vi "期末-6.vi"() -> ()   [LabVIEW 2014]
uses:
  <vilib>/vision/NI_Vision_Development_Module.lvlib
panel:
  in  "紀錄":bool
  out "分量和":dbl[](array[numeric])
  in  "填入飽和磁場分量中點座標":dbl[](array[numeric])
  in  "Stop Button":bool
  out "0. 原始畫面":T1(plugin-control)
  in  "1. 範圍選擇":T2={"色相（H）"={0, 255}, "飽和度（S）"={0, 255}, "亮度（L）"={0, 255}} {"亮度（L）" scale=0.0..255.0; "飽和度（S）" scale=0.0..255.0; "色相（H）" scale=0.0..255.0}
  out "Number of Particles":i32
  out "output cluster":cluster{"X":dbl, "Y":dbl}
  in  "顏色範圍初始化":bool
  in  "Tab Control":T3(tab)
  out "1. 顏色選取":T1(plugin-control)
  out "2. 填補空隙":T1(plugin-control)
  out "4. 形狀修正":T1(plugin-control)
  out "5. 選取結果":T1(plugin-control)
  out "Particle Measurements":dbl[][](array[numeric])
  out "Error Out":errorcluster
  out "瞬間尖點座標":dbl[][](array[numeric])
  out "滑鼠位置顏色":T4
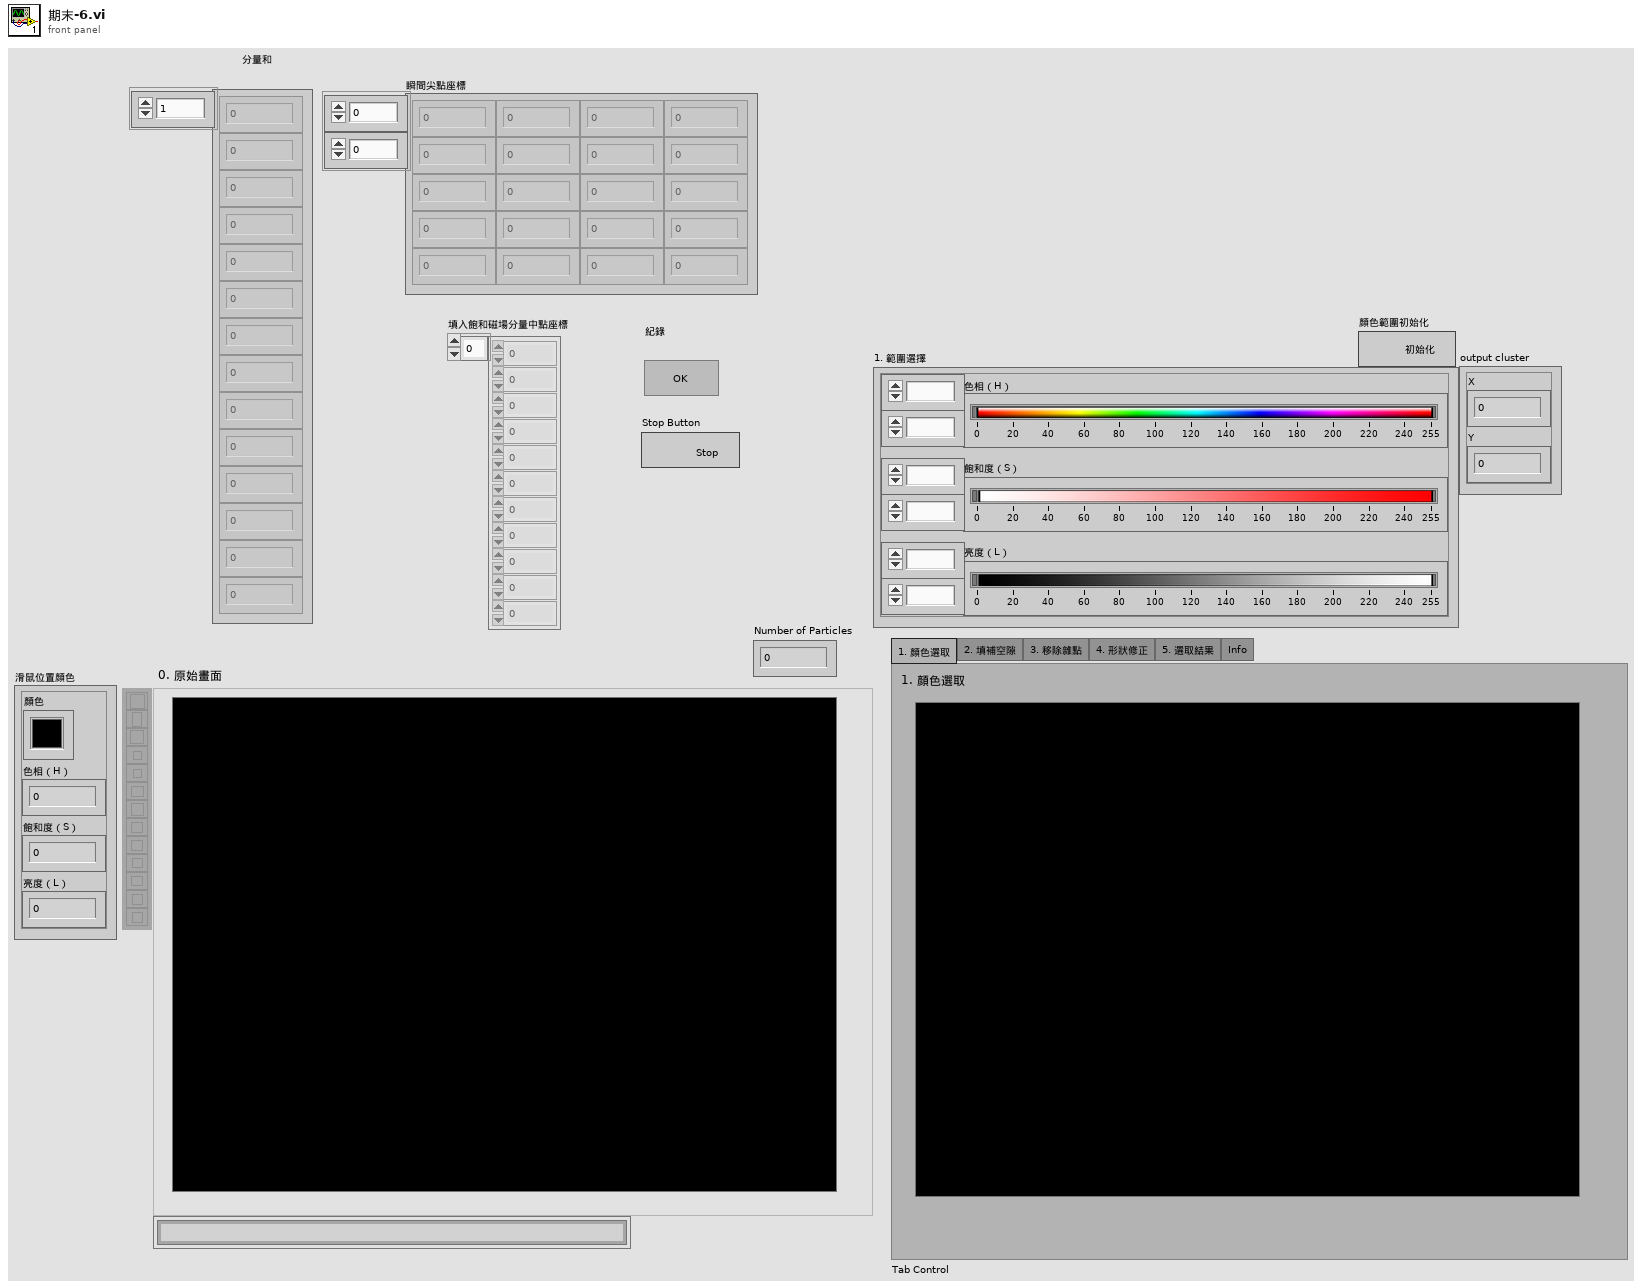
[diagram p1: front panel]
types:
  T1 = typedef "IMAQ Image.ctl" = refnum<image>
  T2 = cluster{"色相（H）":cluster{u8, u8}, "飽和度（S）":cluster{u8, u8}, "亮度（L）":cluster{u8, u8}}
  T3 = enum32{"1. 顏色選取", "2. 填補空隙", "3. 移除雜點", "4. 形狀修正", "5. 選取結果", "Info"}
  T4 = cluster{"色相（H）":u8, "飽和度（S）":u8, "亮度（L）":u8, "顏色":u32}
  T5 = cluster{"Numeric":dbl, "Numeric":dbl, "Numeric":dbl, "Numeric":dbl}
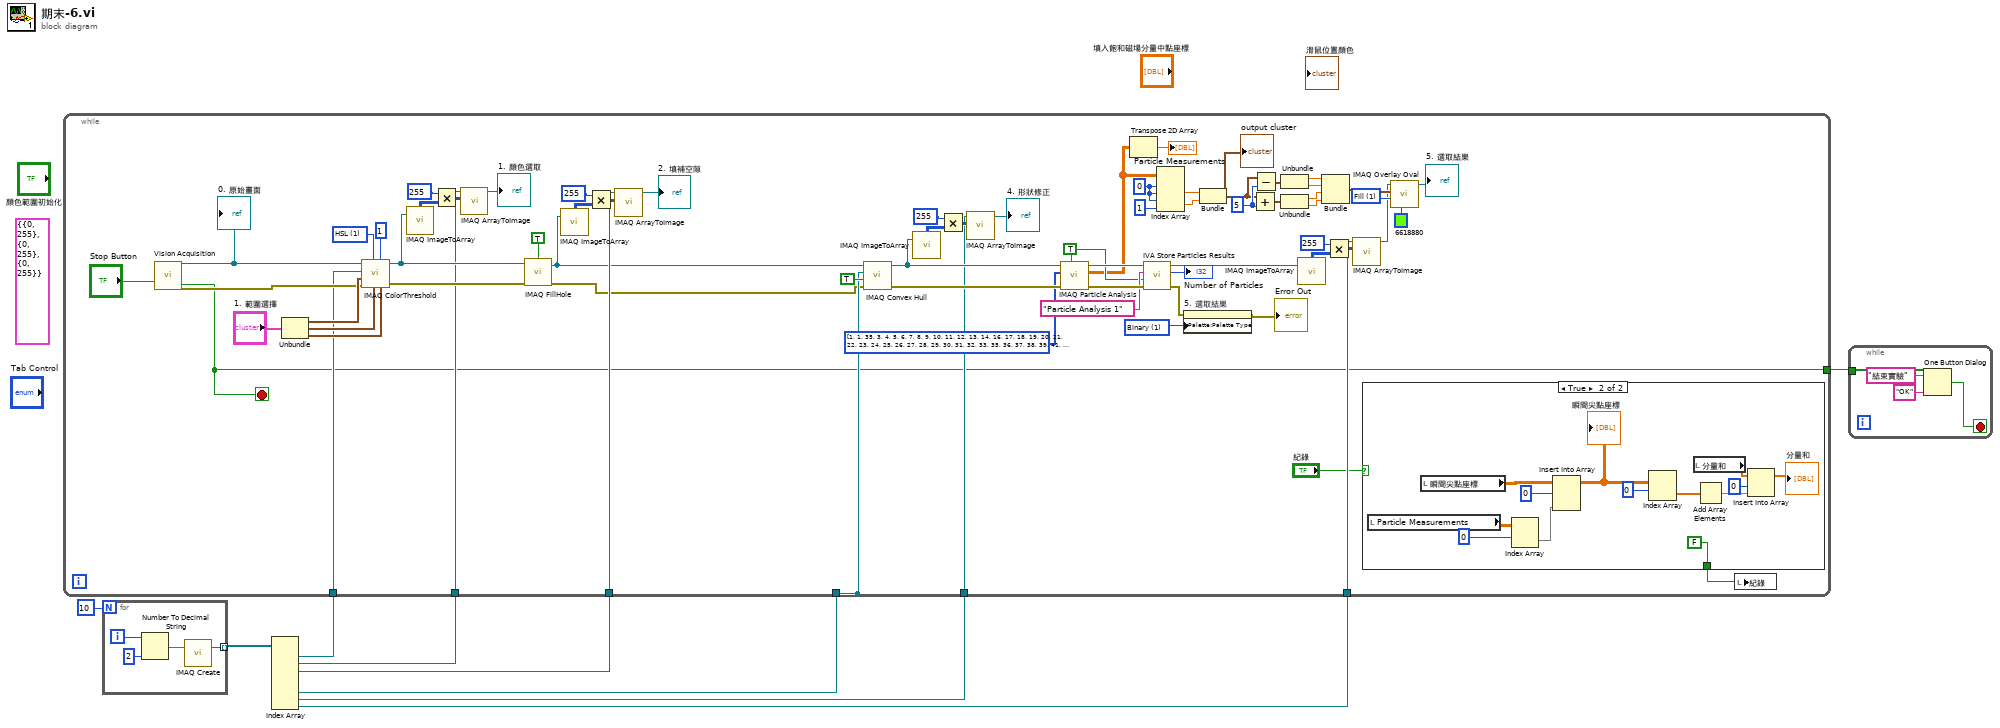
[diagram p0: block diagram]
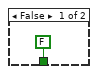
[diagram p2: hidden frame]
diagram:
  (unwired) T2 {"色相（H）"={0, 255}, "飽和度（S）"={0, 255}, "亮度（L）"={0, 255}} ("範圍選擇")
  n1 = for {
    N: 10 -> [_]
    tunnel: [w10] -> w9 mode=indexing
    i -> [w12]
    n2 = Number To Decimal String(number=w12, width (-)=2) -> (decimal integer string=w11:string)
    n3 = call "IMAQ Create"("Image Name"=w11) -> ("New Image"=w10:T1)  [unwired: 4 in, 1 out]
  }
  n4 = Index Array(array=w9) -> (element #1=w8:T1, element #2=w7:T1, element #3=w6:T1, element #6=w4:T1, element #7=w3:T1, element #8=w2:T1)  [unwired: 8 in, 2 out]
  n5 = while {
    tunnel: w6 -> [w52]
    tunnel: w4 -> [w63]
    tunnel: [w63] -> _
    tunnel: w7 -> [w57]
    tunnel: w8 -> [w51]
    tunnel: w3 -> [w45]
    tunnel: w2 -> [w22]
    tunnel: [w16] -> w1
    stop <- w16 stop-if-true
    w27 = u32 1 items=["Frame", "Fill"] ("Drawing Mode (Frame)")
    w36 = 5
    w41 = 0
    w65 = u32 1 items=["Grayscale", "Binary", "Gradient", "Rainbow", "Temperature", "User Defined"] ("Palette")
    w70 = i32[] [1, 1, 35, 3, 4, 5, 6, 7, 8, 9, 10, 11, 12, 13, 14, 16, 17, 18, 19, 20, 21, 22, 23, 24, 25, 26, 27, 28, 29, 30, 31, 32, 33, 35, 36, 37, 38, 39, 41, 42, 43, 45, 46, 48, 49, 50, 51, 53, 54, 55, 56, 58, 59, 60, 61, 62, 63, 64, 65, 66, 68, 69, 70, 71, 72, 73, 74, 75, 76, 77, 78, 79, 80, 81, 82, 83, 84, 85, 86, 87, 88] items=["Center of Mass X", "Center of Mass Y", "First Pixel X", "First Pixel Y", "Bounding Rect Left", "Bounding Rect Top", "Bounding Rect Right", "Bounding Rect Bottom", "Max Feret Diameter Start X", "Max Feret Diameter Start Y", "Max Feret Diameter End X", "Max Feret Diameter End Y", "Max Horiz. Segment Length Left", "Max Horiz. Segment Length Right", "Max Horiz. Segment Length Row", "-", "Bounding Rect Width", "Bounding Rect Height", "Bounding Rect Diagonal", "Perimeter", "Convex Hull Perimeter", "Holes' Perimeter", "Max Feret Diameter", "Equivalent Ellipse Major Axis", "Equivalent Ellipse Minor Axis", "Equivalent Ellipse Minor Axis (Feret)", "Equivalent Rect Long Side", "Equivalent Rect Short Side", "Equivalent Rect Diagonal", "Equivalent Rect Short Side (Feret)", "Average Horiz. Segment Length", "Average Vert. Segment Length", "Hydraulic Radius", "Waddel Disk Diameter", "-", "Area", "Holes' Area", "Particle & Holes' Area", "Convex Hull Area", "Image Area", "-", "Number of Holes", "Number of Horiz. Segments", "Number of Vert. Segments", "-", "Orientation", "Max Feret Diameter Orientation", "-", "% Area/Image Area", "% Area/(Particle & Holes' Area)", "Ratio of Equivalent Ellipse Axes", "Ratio of Equivalent Rect Sides", "-", "Elongation Factor", "Compactness Factor", "Heywood Circularity Factor", "Type Factor", "-", "Sum X", "Sum Y", "Sum XX", "Sum XY", "Sum YY", "Sum XXX", "Sum XXY", "Sum XYY", "Sum YYY", "-", "Moment of Inertia XX", "Moment of Inertia XY", "Moment of Inertia YY", "Moment of Inertia XXX", "Moment of Inertia XXY", "Moment of Inertia XYY", "Moment of Inertia YYY", "Norm. Moment of Inertia XX", "Norm. Moment of Inertia XY", "Norm. Moment of Inertia YY", "Norm. Moment of Inertia XXX", "Norm. Moment of Inertia XXY", "Norm. Moment of Inertia XYY", "Norm. Moment of Inertia YYY", "Hu Moment 1", "Hu Moment 2", "Hu Moment 3", "Hu Moment 4", "Hu Moment 5", "Hu Moment 6", "Hu Moment 7"] ("Pixel Measurements")
    w72 = TRUE ("Connectivity 4/8 (8)")
    w81 = u16 1 items=["RGB", "HSL", "HSV", "HSI"] ("Color Mode")
    n6 = call "Vision Acquisition"("Stop (F)"="Stop Button") -> ("Image Out"=w83:T1, "Stopped"=w16:bool, "error out"=w76:errorcluster)  [unwired: 24 in]
    "0. 原始畫面" <- w83
    n7 = Unbundle("1. 範圍選擇") -> ("色相（H）"=w80:cluster{u8, u8}, "飽和度（S）"=w79:cluster{u8, u8}, "亮度（L）"=w78:cluster{u8, u8})
    n8 = call "IMAQ ColorThreshold"("Blue or Luma or Val or Inten Range"=w78, "Replace Value"=1, "Green or Sat Range"=w79, "Color Mode"=w81, "error in (no error)"=w76, "Red or Hue Range"=w80, "Image Dst"=w51, "Image Src"=w83) -> ("error out"=w67:errorcluster, "Image Dst Out"=w62:T1)  [unwired: 2 out]
    n9 = call "IMAQ ImageToArray"("Image"=w62) -> ("Image Pixels (U8)"=w60:u8[][])  [unwired: 3 in, 4 out]
    n10 = Multiply(x=255, y=w60) -> (x*y=w59:i32[][])
    n11 = call "IMAQ ArrayToImage"("Image Pixels (U8)"=w59, "Image"=w57) -> ("Image Out"=→"1. 顏色選取":T1)  [unwired: 8 in, 1 out]
    n12 = call "IMAQ FillHole"("error in (no error)"=w67, "Image Src"=w62, "Connectivity 4/8 (8)"=TRUE) -> ("error out"=w14:errorcluster, "Image Dst Out"=w15:T1)  [unwired: 1 in, 2 out]
    n13 = call "IMAQ ImageToArray"("Image"=w15) -> ("Image Pixels (U8)"=w55:u8[][])  [unwired: 3 in, 4 out]
    n14 = Multiply(x=255, y=w55) -> (x*y=w56:i32[][])
    n15 = call "IMAQ ArrayToImage"("Image Pixels (U8)"=w56, "Image"=w52) -> ("Image Out"=→"2. 填補空隙":T1)  [unwired: 8 in, 1 out]
    n16 = call "IMAQ Convex Hull"("error in (no error)"=w14, "Connectivity 4/8 (8)"=TRUE, "Image Dst"=w63, "Image Src"=w15) -> ("error out"=w71:errorcluster, "Image Dst Out"=w46:T1)  [unwired: 6 out]
    n17 = call "IMAQ ImageToArray"("Image"=w46) -> ("Image Pixels (U8)"=w49:u8[][])  [unwired: 3 in, 4 out]
    n18 = Multiply(x=255, y=w49) -> (x*y=w50:i32[][])
    n19 = call "IMAQ ArrayToImage"("Image Pixels (U8)"=w50, "Image"=w45) -> ("Image Out"=→"4. 形狀修正":T1)  [unwired: 8 in, 1 out]
    n20 = call "IMAQ Particle Analysis"("Connectivity 4/8 (8)"=w72, "error in (no error)"=w71, "Pixel Measurements"=w70, "Image"=w46) -> ("error out"=w75:errorcluster, "Particle Measurements (Pixels)"=w42:dbl[][], "Image Out (duplicate)"=w73:T1)  [unwired: 1 in, 4 out]
    n21 = Transpose 2D Array(2D array=w42) -> (transposed array=→"Particle Measurements":dbl[][])
    n22 = call <vilib>:"IVA Store Particles Results.vi"("error in (no error)"=w75, "Connectivity 4/8 (8)"=w72, "Step Name"="Particle Analysis 1", "Image in"=w73) -> ("error out"=w66:errorcluster, "Number of Particles"=→"Number of Particles":i32, "Image dup"=w26:T1)  [unwired: 5 out]
    n23 = Index Array(array=w42, index (row) #1=w41, index (col) #1=w41, index (row) #2=w41, index (col) #2=1) -> (element #1=w39:dbl, element #2=w38:dbl)
    n24 = property on="5. 選取結果" class="ImageControl"(error in=w66, "Palette:Palette Type"=w65) -> (error out=→"Error Out":errorcluster)  [unwired: 1 in, 1 out]
    n25 = Bundle("Numeric"=w39, "Numeric"=w38) -> (w35:cluster{"Numeric":dbl, "Numeric":dbl})  [unwired: 1 in]
    "output cluster" <- w35
    n26 = Add(x=w35, y=w36) -> (x+y=w33:cluster{"Numeric":dbl, "Numeric":dbl})
    n27 = Subtract(x=w35, y=w36) -> (x-y=w34:cluster{"Numeric":dbl, "Numeric":dbl})
    n28 = Unbundle(w34) -> ("Numeric"=w32:dbl, "Numeric"=w31:dbl)
    n29 = Unbundle(w33) -> ("Numeric"=w30:dbl, "Numeric"=w29:dbl)
    n30 = call "IMAQ ImageToArray"("Image"=w26) -> ("Image Pixels (U8)"=w23:u8[][])  [unwired: 3 in, 4 out]
    n31 = Bundle("Numeric"=w32, "Numeric"=w31, "Numeric"=w30, "Numeric"=w29) -> (w28:T5)  [unwired: 1 in]
    n32 = Multiply(x=255, y=w23) -> (x*y=w24:i32[][])
    n33 = call "IMAQ ArrayToImage"("Image Pixels (U8)"=w24, "Image"=w22) -> ("Image Out"=w21:T1)  [unwired: 8 in, 1 out]
    n34 = case shown="True" "紀錄" {
      tunnel: [FALSE FALSE] -> w17
      frame False {
      }
      frame True {
        n35 = local read "Particle Measurements"() -> (w87:dbl[][])
        n36 = local read "瞬間尖點座標"() -> (w93:dbl[][])
        n37 = Index Array(array=w87, index (row)=0) -> (element=w92:dbl[])  [unwired: 1 in]
        n38 = Insert Into Array(array=w93, index (row)=0 ("index"), new element=w92) -> (w95:dbl[][])  [unwired: 1 in]
        "瞬間尖點座標" <- w95
        n39 = Index Array(array=w95, index (row)=0) -> (element=w97:dbl[])  [unwired: 1 in]
        n40 = local read "分量和"() -> (w88:dbl[])
        n41 = Add Array Elements(numeric array=w97) -> (sum=w90:dbl)
        n42 = Insert Into Array(array=w88, index=0 ("index (row)"), new element=w90) -> (→"分量和":dbl[])
      }
    }
    n43 = call "IMAQ Overlay Oval"("Color"=u32 6618880, "Drawing Mode (Frame)"=w27, "Bounding Rectangle"=w28, "Image"=w21) -> ("Image Out"=→"5. 選取結果":T1)  [unwired: 6 in, 1 out]
    n44 = local write "紀錄"(w17) -> ()
  }
  n45 = while {
    tunnel: w1 -> [_]
    stop <- w100 stop-if-true
    n46 = One Button Dialog(message="結束實驗", button name ("OK")="OK") -> (true=w100:bool)
  }
